vi "GetFrontPanel.vi"(8 "ErrorIn":errorcluster, 11 "ReferenceIn":refnum<class "VerticalButtonBar.lvclass">) -> (0 "ErrorOut":errorcluster, 2 "FrontPanel":refnum<class "FrontPanelControl.lvclass">, 3 "ReferenceIn":refnum<class "VerticalButtonBar.lvclass">)   [LabVIEW 2021, in "VerticalButtonBar.lvclass"]
doc: "Retrieve the FrontPanelControl for controlling the state of the user interface front panel"
uses:
  VerticalButtonBar.lvclass
  Library_UserInterface_FrontPanelControl/FrontPanelControl/FrontPanelControl.lvclass
  VerticalButtonBar.lvclass/VerticalButtonBar.ctl
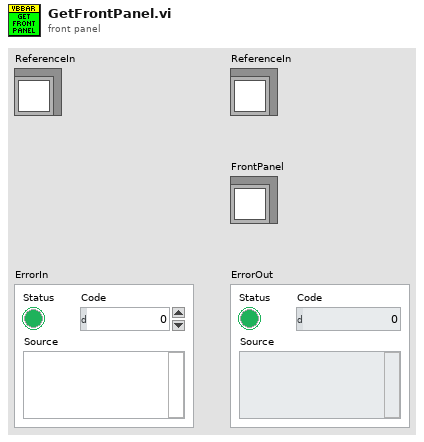
[diagram p1: front panel]
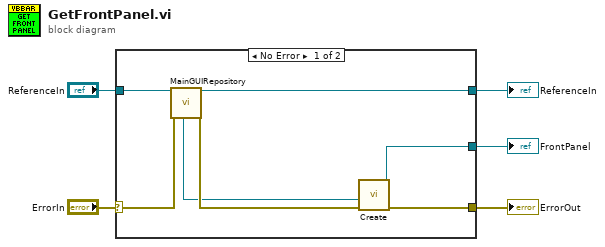
[diagram p0: block diagram]
diagram:
  n1 = case shown="No Error" "ErrorIn" {
    selector: "ErrorIn" -> [w12 w14]
    tunnel: [w10 w14] -> w4
    tunnel: [w8 w13] -> w2
    tunnel: "ReferenceIn" -> [w9 w13]
    tunnel: [w6 _] -> w1
    frame No Error {
      n2 = call "MainGUIRepository.vi"("ReferenceIn"=w9, "ErrorIn"=w12) -> ("ProcessViRef"=w7:refnum<vi>, "ReferenceOut"=w8:refnum<class "VerticalButtonBar.lvclass">, "ErrorOut"=w11:errorcluster)  [unwired: 10 in, 5 out]
      n3 = call "Create.vi"("ErrorIn"=w11, "VIRef"=w7) -> ("ErrorOut"=w10:errorcluster, "ObjectOut"=w6:refnum<class "FrontPanelControl.lvclass">)  [unwired: 8 in]
    }
    frame Error {
    }
  }
  "ErrorOut" <- w4
  "ReferenceIn" <- w2
  "FrontPanel" <- w1
